vi "Running Histogram.vi"(6 "重置":bool, 8 "区间":i32=20, 9 "最大值":dbl=10.0 format="%0.2f", 10 "最小值":dbl=-10.0 format="%0.2f", 11 "输入数据":dbl[](array[numeric])) -> (1 "总计数":i32, 2 "X轴":dbl[](array[numeric]), 3 "直方图":dbl[](array[numeric]), 4 "超出范围":cluster{"过低计数":i32, "过高计数":i32})   [LabVIEW 2012]
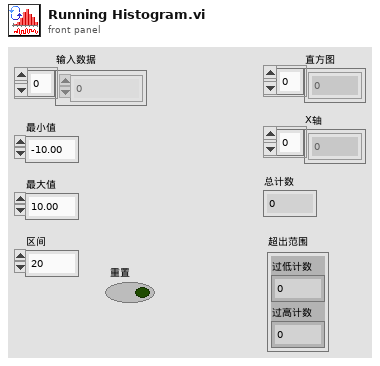
[diagram p1: front panel]
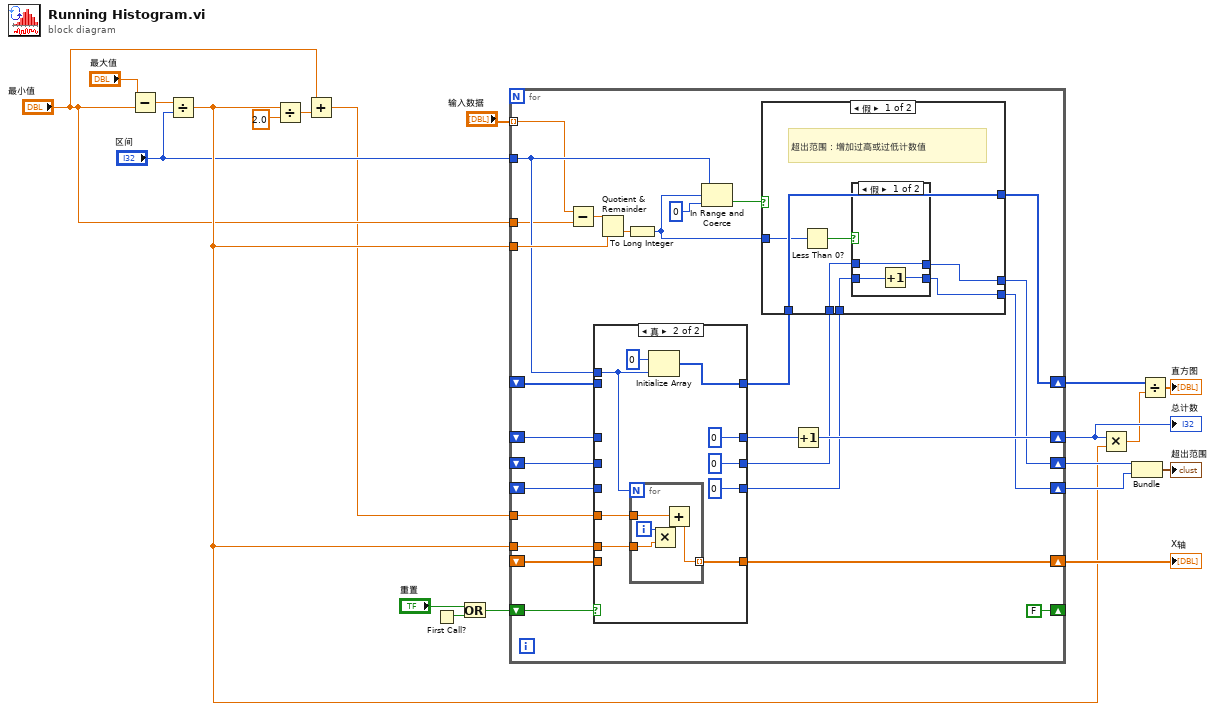
[diagram p0: block diagram]
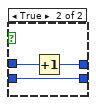
[diagram p3: hidden frame]
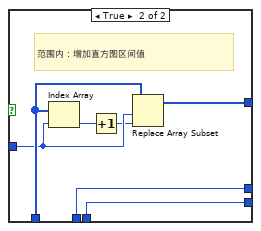
[diagram p4: hidden frame]
diagram:
  n1 = Subtract ("减")(x="最大值", y="最小值") -> (x-y=w4:dbl)
  n2 = Divide ("除")(x=w4, y="区间") -> (x/y=w7:dbl)
  n3 = Divide ("除")(x=w7, y=2.0) -> (x/y=w2:dbl)
  n4 = Add ("加")(x="最小值", y=w2) -> (x+y=w1:dbl)
  n5 = First Call? ("首次调用？")() -> (First Call?: T/F=w20:bool)
  n6 = Or ("或")(x="重置", y=w20) -> (x .or. y?=w18:bool)
  n7 = for {
    tunnel: "输入数据" -> [w40] mode=indexing
    tunnel: "最小值" -> [w25]
    tunnel: w7 -> [w46]
    tunnel: "区间" -> [w41]
    shift-right: [w35] -> w15
    shift-left: _ -> [w39]
    shift-right: [w29] -> w11
    shift-left: _ -> [w38]
    shift-right: [w30] -> w10
    shift-left: _ -> [w37]
    shift-right: [w27] -> w17
    shift-left: _ -> [w34]
    shift-right: [FALSE] -> _
    shift-left: w18 -> [w42]
    tunnel: w1 -> [w24]
    tunnel: w7 -> [w23]
    shift-right: [w21] -> w12
    shift-left: _ -> [w22]
    n8 = Subtract ("减")(x=w40, y=w25) -> (x-y=w47:dbl)
    n9 = case shown="真" w42 {
      tunnel: w41 -> [_ w53]
      tunnel: [w52 0 ("元素")] -> w36
      tunnel: [w51 0 ("元素")] -> w32
      tunnel: [w50 0 ("元素")] -> w31
      tunnel: w39 -> [w52 _]
      tunnel: w38 -> [w51 _]
      tunnel: w37 -> [w50 _]
      tunnel: [w49 w57] -> w28
      tunnel: w34 -> [w49 _]
      tunnel: w24 -> [_ w56]
      tunnel: w23 -> [_ w55]
      tunnel: w22 -> [w48 _]
      tunnel: [w48 w54] -> w21
      frame False {
      }
      frame True {
        n10 = for {
          N: w53 -> [_]
          tunnel: w56 -> [w66]
          tunnel: w55 -> [w64]
          tunnel: [w62] -> w54 mode=indexing
          i -> [w65]
          n11 = Multiply ("乘")(x=w65, y=w64) -> (x*y=w63:dbl)
          n12 = Add ("加")(x=w66, y=w63) -> (x+y=w62:dbl)
        }
        n13 = Initialize Array ("初始化数组")(0 ("元素"), w53) -> (w57:i32[])
      }
    }
    n14 = Quotient & Remainder ("商与余数")(x=w47, y=w46) -> (floor(x/y)=w43:dbl)  [unwired: 1 out]
    n15 = To Long Integer ("转换为长整型")(number=w43) -> (32bit integer=w26:i32)
    n16 = In Range and Coerce ("判定范围并强制转换")(upper limit=w41, x=w26, lower limit=0 ("下限")) -> (In Range?=w44:bool)  [unwired: 1 out]
    n17 = case shown="假" w44 {
      tunnel: w32 -> [w72 w81]
      tunnel: w31 -> [w71 w80]
      tunnel: [w70 w81] -> w29
      tunnel: [w69 w80] -> w30
      tunnel: w28 -> [w68 w85]
      tunnel: [w68 w82] -> w27
      tunnel: w26 -> [w67 w84]
      frame False {
        # "超出范围：增加过高或过低计数值"
        n18 = Less Than 0? ("小于0？")(x=w67) -> (x < 0?=w73:bool)
        n19 = case shown="假" w73 {
          tunnel: w72 -> [w74 w79]
          tunnel: w71 -> [w75 w77]
          tunnel: [w74 w78] -> w70
          tunnel: [w76 w77] -> w69
          frame False {
            n20 = Increment ("加1")(x=w75) -> (x+1=w76:i32)
          }
          frame True {
            n21 = Increment ("加1")(x=w79) -> (x+1=w78:i32)
          }
        }
      }
      frame True {
        # "范围内：增加直方图区间值"
        n22 = Index Array ("索引数组")(array=w85, index=w84) -> (element=w86:i32)
        n23 = Increment ("加1")(x=w86) -> (x+1=w83:i32)
        n24 = Replace Array Subset ("替换数组子集")(array=w85, new element=w83, index=w84) -> (w82:i32[])
      }
    }
    n25 = Increment ("加1")(x=w36) -> (x+1=w35:i32)
  }
  "总计数" <- w15
  "X轴" <- w12
  n26 = Multiply ("乘")(x=w15, y=w7) -> (x*y=w14:dbl)
  n27 = Bundle ("捆绑")("元素"=w11, "元素"=w10) -> (→"超出范围":cluster{"元素":i32, "元素":i32})  [unwired: 1 in]
  n28 = Divide ("除")(x=w17, y=w14) -> (x/y=→"直方图":dbl[])
